vi "ID号显示.vi"(11 "输入数组":u8[](array[numeric]) format="%x") -> (3 "输出字符串":string)   [LabVIEW 2015]
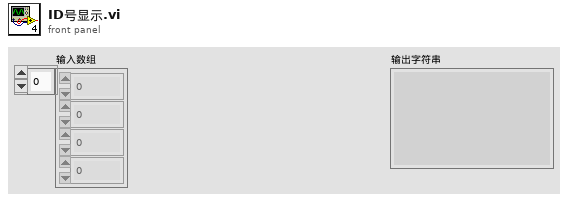
[diagram p1: front panel]
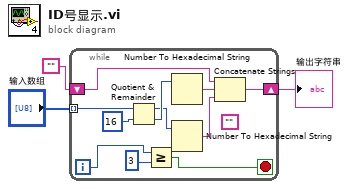
[diagram p0: block diagram]
diagram:
  n1 = while {
    tunnel: "输入数组" -> [w14] mode=indexing
    shift-right: [w11] -> w3
    shift-left: "" -> [w12]
    i -> [w6]
    stop <- w4 stop-if-true
    (unwired) ""
    n2 = Quotient & Remainder(x=w14, y=u8 16) -> (x-y*floor(x/y)=w9:u8, floor(x/y)=w10:u8)
    n3 = Greater Or Equal?(x=w6, y=u8 3) -> (x >= y?=w4:bool)
    n4 = Number To Hexadecimal String(2:w10) -> (0:w7:string)  [unwired: 1 in]
    n5 = Number To Hexadecimal String(2:w9) -> (0:w8:string)  [unwired: 1 in]
    n6 = Concatenate Strings(w12, w7, w8) -> (w11:string)
  }
  "输出字符串" <- w3
